vi "Read Parameter.vi"(8 "error in (no error)":errorcluster caption="错误输入（无错误）") -> (0 "错误输出":errorcluster, 2 "Param Out":T1)   [LabVIEW 2023]
uses:
  Ctl/Global Parameter.ctl
  <vilib>/Utility/xml.llb/Read From XML File(string).vi
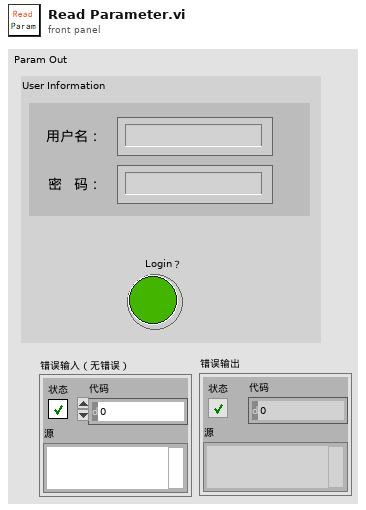
[diagram p1: front panel]
types:
  T1 = typedef "Global Parameter.ctl" = cluster{"User Information":cluster{"用户名：":string, "密   码：":string}, "Login？":bool}
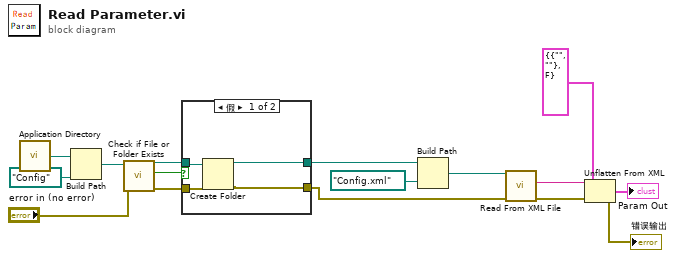
[diagram p0: block diagram]
diagram:
  n1 = call <vilib>:"Application Directory.vi"() -> ("Application Directory"=w16:path)
  n2 = Build Path(base path=w16, name or relative path=path "Config" ("名称或相对路径")) -> (appended path=w14:path)
  n3 = call <vilib>:"Check if File or Folder Exists.vi"("error in (no error)"="error in (no error)", "path"=w14) -> ("error out"=w11:errorcluster, "file or folder exists?"=w13:bool, "dup path"=w12:path)  [unwired: 7 in]
  n4 = case shown="假" w13 {
    tunnel: w12 -> [w20 w22]
    tunnel: w11 -> [w19 w21]
    tunnel: [w18 w21] -> w3
    tunnel: [w17 w22] -> w10
    frame False {
      n5 = Create Folder(path (use dialog)=w20, error in=w19) -> (created path=w17:path, error out=w18:errorcluster)  [unwired: 1 in, 1 out]
    }
    frame True {
    }
  }
  n6 = Build Path(base path=w10, name or relative path=path "Config.xml" ("名称或相对路径")) -> (appended path=w8:path)
  n7 = call-poly <vilib>:"Read From XML File.vi"("error in (no error)"=w3, "XML File Path"=w8) -> ("error out"=w2:errorcluster, "XML Elements"=w7:string)  [unwired: 7 in, 1 out]
  n8 = Unflatten From XML(xml string=w7, type=T1 {"User Information"={"用户名："="", "密   码："=""}, "Login？"=FALSE} ("Write"), error in (no error)=w2) -> (value=→"Param Out":T1, error out=→"错误输出":errorcluster)
